vi "Poll Sample Container.vi"(8 "error in (no error)":errorcluster, 10 "Sample Container":T1, 11 "CO2 Actor in":refnum<class "CO2 Actor.lvclass">) -> (0 "error out":errorcluster)   [LabVIEW 2015, in "cRIO-Carbondioxide.lvlib" / "CO2-Actor.lvlib" / "CO2 Actor.lvclass"]
uses:
  CO2 Actor.lvclass
  Controls/Sample Container.ctl
  subs/Sample/Sample.lvclass
  <vilib>/ActorFramework/Actor/Actor.lvclass/Actor.ctl
  <vilib>/ActorFramework/Message Enqueuer/Message Enqueuer.lvclass/Message Enqueuer.ctl
  CO2 Actor Messages/Check Sample Container Msg/Check Sample Container Msg.lvclass/Check Sample Container Msg.ctl
  <vilib>/ActorFramework/Message Enqueuer/Enqueue.vi
  <vilib>/ActorFramework/Actor/Read Self Enqueuer.vi
  <vilib>/ActorFramework/Message Enqueuer/Init from Existing Queue.vi
  <vilib>/ActorFramework/Message Priority Queue/Priority Enqueue.vi
  CO2 Actor Messages/Check Sample Container Msg/Check Sample Container Msg.lvclass
  <vilib>/ActorFramework/Message Enqueuer/Message Enqueuer.lvclass
  <vilib>/ActorFramework/Actor/Actor.lvclass
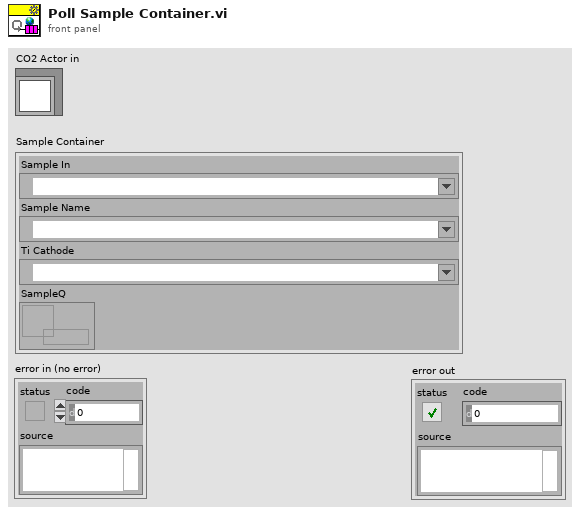
[diagram p1: front panel]
types:
  T1 = typedef "Sample Container.ctl" = cluster{"Sample In":refnum<k21>, "Sample Name":refnum<k21>, "Ti Cathode":refnum<k21>, "SampleQ":refnum<queue>}
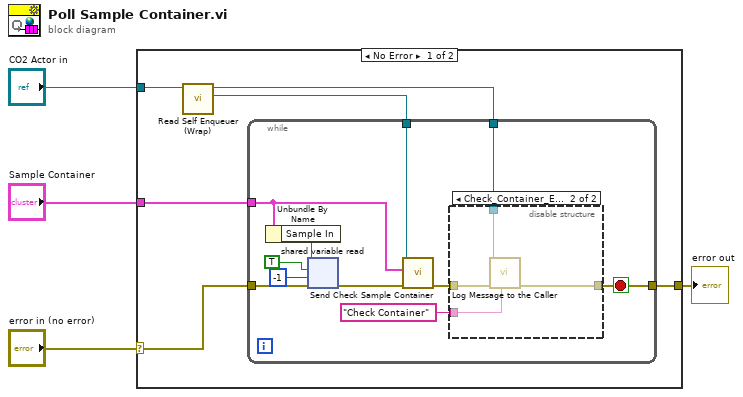
[diagram p0: block diagram]
diagram:
  n1 = case shown="No Error" "error in (no error)" {
    selector: "error in (no error)" -> [w9 w27]
    tunnel: "CO2 Actor in" -> [w7 _]
    tunnel: "Sample Container" -> [w10 _]
    tunnel: [w8 w27] -> w1
    frame No Error {
      n2 = call "Read Self Enqueuer (Wrap).vi"("CO2 Actor in"=w7) -> ("Actor Framework:Message Enqueuer"=w6:refnum<class "Message Enqueuer.lvclass">, "CO2 Actor out"=w5:refnum<class "CO2 Actor.lvclass">)  [unwired: 9 in]
      n3 = while {
        tunnel: w10 -> [w11]
        tunnel: w9 -> [w18]
        tunnel: [w15] -> w8
        tunnel: w6 -> [w17]
        tunnel: w5 -> [w16]
        stop <- w15 stop-if-true
        n4 = Unbundle By Name(w11) -> ("Sample In"=w21:refnum<k21>)
        n5 = shared-variable-read(w21, w18, TRUE, -1 ("timeout ms")) -> (w12:errorcluster)  [unwired: 4 out]
        n6 = call "Send Check Sample Container.vi"("error in (no error)"=w12, "Sample Container"=w11, "Message Enqueuer"=w17) -> ("error out"=w14:errorcluster)  [unwired: 7 in, 1 out]
        n7 = disable-structure shown="Check_Container_Echo==ON" {
          disable-tunnel: w16 -> [_ w24]
          disable-tunnel: [w22 w25] -> w15
          disable-tunnel: w14 -> [w22 w26]
          disable-tunnel: "Check Container" ("String (\"\" = no message to send)") -> [_ w23]
          frame condition #0 (active) {
          }
          frame condition #1 {
            n8 = call-dynamic "Log Message to the Caller.vi"("String (\"\" = no message to send)"=w23, "error in (no error)"=w26, "CO2 Actor in"=w24) -> ("error out"=w25:errorcluster)  [unwired: 7 in, 1 out]
          }
        }
      }
    }
    frame Error {
    }
  }
  "error out" <- w1
